vi "Ex4 christo.vi"() -> ()   [LabVIEW 2018]
panel:
  out "?":bool
  out "?":bool
  out "?":bool
  out "?":bool
  out "?":bool
  out "?":bool
  out "?":bool
  in  "Chiffre":i8=1 min=1 max=6
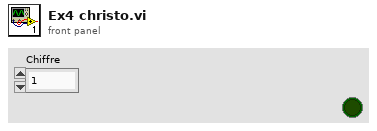
[diagram p1: front panel]
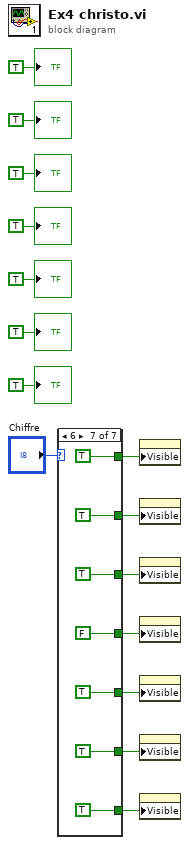
[diagram p0: block diagram]
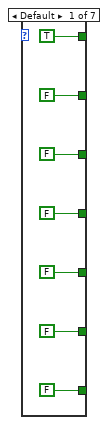
[diagram p2: hidden frame]
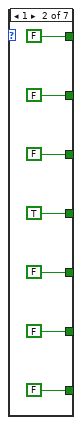
[diagram p3: hidden frame]
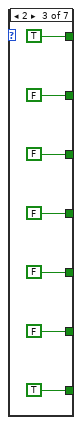
[diagram p4: hidden frame]
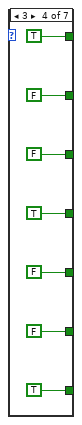
[diagram p5: hidden frame]
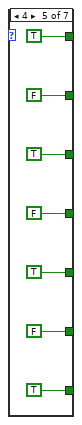
[diagram p6: hidden frame]
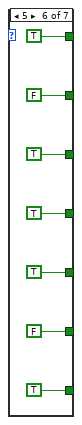
[diagram p7: hidden frame]
diagram:
  n1 = case shown="6" "Chiffre" {
    tunnel: [FALSE ("Visible") FALSE ("Visible") FALSE ("Visible") FALSE ("Visible") FALSE ("Visible") FALSE ("Visible") TRUE ("Visible")] -> w15
    tunnel: [TRUE ("Visible") FALSE ("Visible") TRUE ("Visible") TRUE ("Visible") TRUE ("Visible") TRUE ("Visible") TRUE ("Visible")] -> w14
    tunnel: [FALSE ("Visible") FALSE ("Visible") FALSE ("Visible") FALSE ("Visible") TRUE ("Visible") TRUE ("Visible") TRUE ("Visible")] -> w13
    tunnel: [FALSE ("status") TRUE ("status") FALSE ("status") TRUE ("status") FALSE ("status") TRUE ("status") FALSE ("status")] -> w12
    tunnel: [FALSE ("Visible") FALSE ("Visible") FALSE ("Visible") FALSE ("Visible") TRUE ("Visible") TRUE ("Visible") TRUE ("Visible")] -> w11
    tunnel: [FALSE ("Visible") FALSE ("Visible") TRUE ("Visible") TRUE ("Visible") TRUE ("Visible") TRUE ("Visible") TRUE ("Visible")] -> w10
    tunnel: [FALSE ("Visible") FALSE ("Visible") FALSE ("Visible") FALSE ("Visible") FALSE ("Visible") FALSE ("Visible") TRUE ("Visible")] -> w8
    frame Default {
    }
    frame 1 {
    }
    frame 2 {
    }
    frame 3 {
    }
    frame 4 {
    }
    frame 5 {
    }
    frame 6 {
    }
  }
  n2 = property class="Bool (strict)"("Visible"=w14) -> ()  [unwired: 2 in, 2 out]
  n3 = property class="Bool (strict)"("Visible"=w8) -> ()  [unwired: 2 in, 2 out]
  n4 = property class="Bool (strict)"("Visible"=w13) -> ()  [unwired: 2 in, 2 out]
  n5 = property class="Bool (strict)"("Visible"=w12) -> ()  [unwired: 2 in, 2 out]
  n6 = property class="Bool (strict)"("Visible"=w11) -> ()  [unwired: 2 in, 2 out]
  n7 = property class="Bool (strict)"("Visible"=w15) -> ()  [unwired: 2 in, 2 out]
  n8 = property class="Bool (strict)"("Visible"=w10) -> ()  [unwired: 2 in, 2 out]
  "?" <- TRUE
  "?" <- TRUE
  "?" <- TRUE
  "?" <- TRUE
  "?" <- TRUE
  "?" <- TRUE
  "?" <- TRUE
